vi "DrawCircle.vi"(1 "Resolution (numPoints)":u32=360, 2 "YCenter":dbl, 3 "XCenter":dbl, 4 "Radius":dbl) -> (0 "Points":cluster{"X":dbl[], "Y":dbl[]})   [LabVIEW 2017, in "ArgosLib.lvlib"]
uses:
  ArgosLib.lvlib
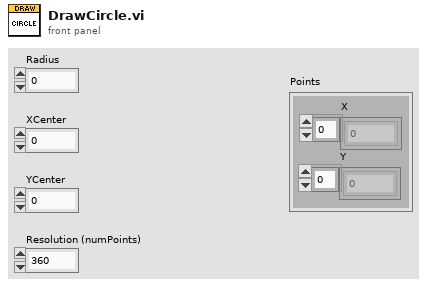
[diagram p1: front panel]
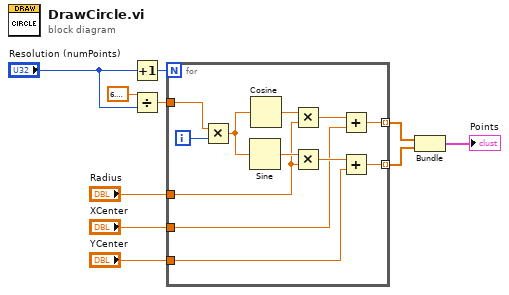
[diagram p0: block diagram]
diagram:
  n1 = Increment(x="Resolution (numPoints)") -> (x+1=w10:u32)
  n2 = Divide(x=6.283185307179586, y="Resolution (numPoints)") -> (x/y=w6:dbl)
  n3 = for {
    N: w10 -> [_]
    tunnel: w6 -> [w22]
    tunnel: "Radius" -> [w17]
    tunnel: "XCenter" -> [w14]
    tunnel: "YCenter" -> [w13]
    tunnel: [w12] -> w2 mode=indexing
    tunnel: [w11] -> w1 mode=indexing
    i -> [w21]
    n4 = Multiply(x=w22, y=w21) -> (x*y=w20:dbl)
    n5 = Sine(x=w20) -> (sin(x)=w19:dbl)
    n6 = Cosine(x=w20) -> (cos(x)=w18:dbl)
    n7 = Multiply(x=w18, y=w17) -> (x*y=w16:dbl)
    n8 = Multiply(x=w19, y=w17) -> (x*y=w15:dbl)
    n9 = Add(x=w16, y=w14) -> (x+y=w12:dbl)
    n10 = Add(x=w15, y=w13) -> (x+y=w11:dbl)
  }
  n11 = Bundle(w2, w1) -> (→"Points":cluster{dbl[], dbl[]})  [unwired: 1 in]
